vi "SetEncPol.vi"(8 "错误输入（无错误）":errorcluster, 10 "编码器序号":i32, 11 "滤波器系数":u8) -> (0 "错误输出":errorcluster)   [LabVIEW 2014]
uses:
  X86Dll/ZXUTConfigMgr.dll
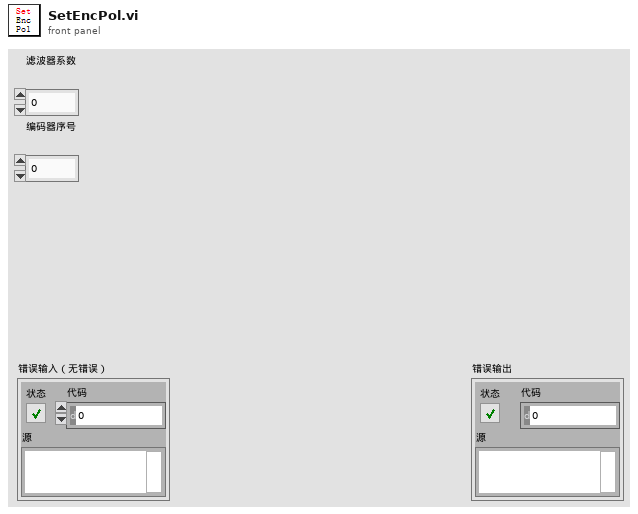
[diagram p1: front panel]
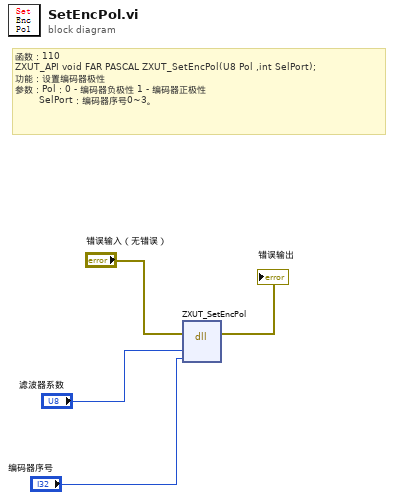
[diagram p0: block diagram]
diagram:
  # "函数：110\nZXUT_API void\tFAR PASCAL ZXUT_SetEncPol(U8 Pol ,int SelPort);\n功能：设置编码器极性\n参数：Pol：0 - 编码器负极性 1 - 编码器正极性\n        SelPort：编码器序号0~3。"
  n1 = dll-call lib="D:/Software/Utrasonic on-line monitoring/X86Dll/ZXUTConfigMgr.dll" fn="ZXUT_SetEncPol"(error in="错误输入（无错误）", "Pol"="滤波器系数", "SelPort"="编码器序号") -> (error out=→"错误输出":errorcluster)  [unwired: 5 in, 1 out]
